vi "Get Temperature.vi"(0 "ICM Ref In":refnum<class "Modbus Master.lvclass">, 11 "error in (no error)":errorcluster) -> (4 "ICM Ref Out":refnum<class "Modbus Master.lvclass">, 6 "Temperature °C":dbl, 15 "error out":errorcluster)   [LabVIEW 2024]
uses:
  <vilib>/NI/Modbus Library/API/Master/Modbus Master.lvclass
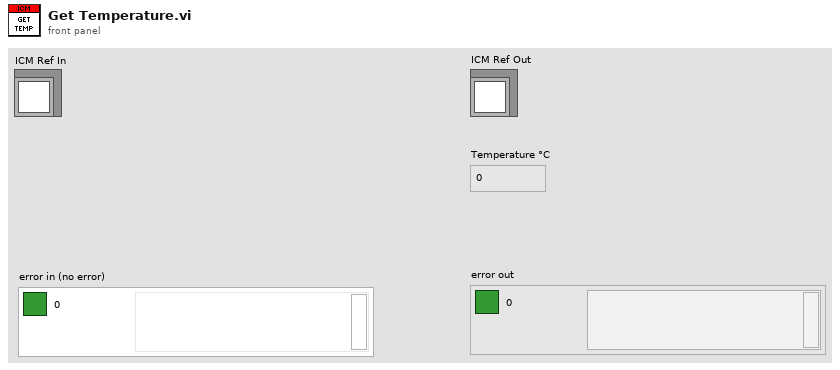
[diagram p1: front panel]
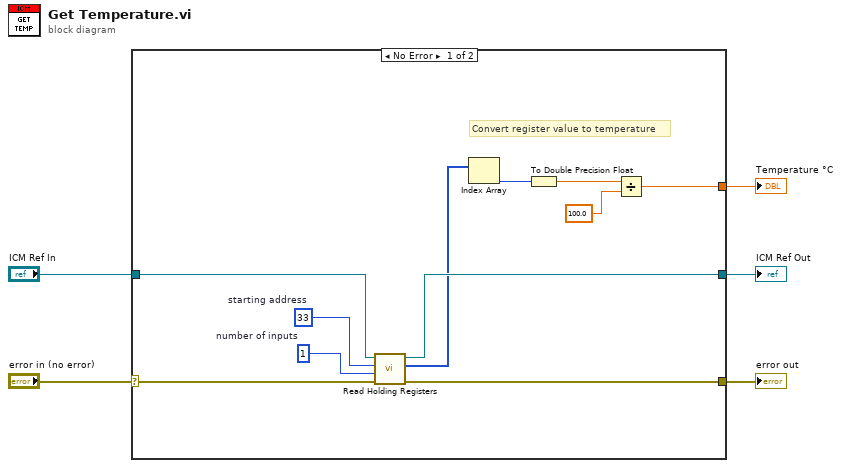
[diagram p0: block diagram]
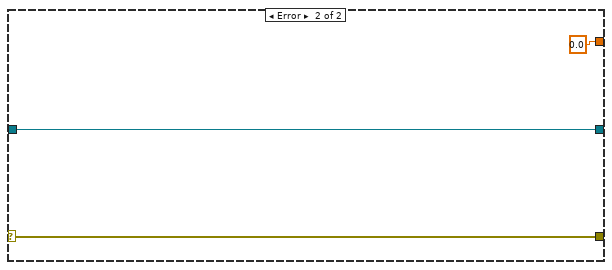
[diagram p2: hidden frame]
diagram:
  n1 = case shown="No Error" "error in (no error)" {
    selector: "error in (no error)" -> [w16 w18]
    tunnel: [w15 w18] -> w5
    tunnel: "ICM Ref In" -> [w14 w19]
    tunnel: [w11 w19] -> w2
    tunnel: [w7 0.0] -> w1
    frame No Error {
      w12 = u16 1  # number of inputs
      w13 = u16 33  # starting address
      # "Convert register value to temperature"
      n2 = call-dynamic "Read Holding Registers.vi"("error in"=w16, "number of inputs"=w12, "starting address"=w13, "Modbus master in"=w14) -> ("error out"=w15:errorcluster, "register values"=w10:u16[], "Modbus master out"=w11:refnum<class "Modbus Master.lvclass">)  [unwired: 5 in]
      n3 = Index Array(array=w10) -> (element=w9:u16)  [unwired: 1 in]
      n4 = To Double Precision Float(number=w9) -> (double precision float=w6:dbl)
      n5 = Divide(x=w6, y=100.0) -> (x/y=w7:dbl)
    }
    frame Error {
    }
  }
  "error out" <- w5
  "ICM Ref Out" <- w2
  "Temperature °C" <- w1
